vi "Resp.vi"(6 "Array 6":string[][](array[string]), 7 "Array":string[][](array[string]), 8 "Array 5":string[][](array[string]), 9 "Array 4":string[][](array[string]), 10 "Array 3":string[][](array[string]), 11 "Array 2":string[][](array[string])) -> (3 "output cluster":T1)   [LabVIEW 2014]
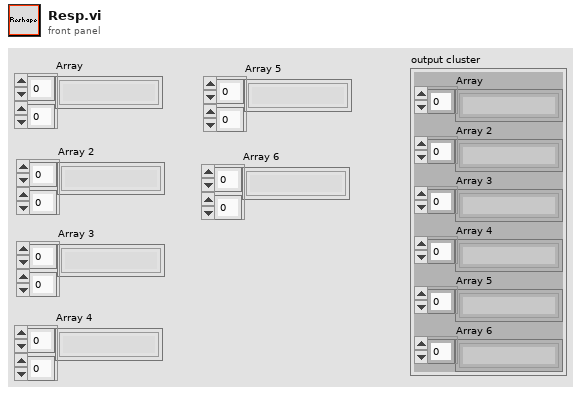
[diagram p1: front panel]
types:
  T1 = cluster{"Array":string[], "Array 2":string[], "Array 3":string[], "Array 4":string[], "Array 5":string[], "Array 6":string[]}
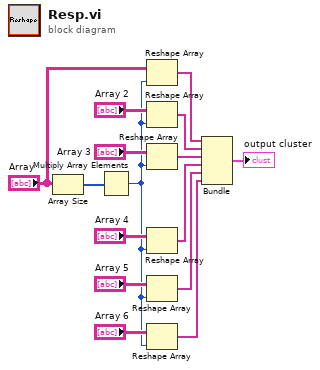
[diagram p0: block diagram]
diagram:
  n1 = Array Size(array="Array") -> (size(s)=w3:i32[])
  n2 = Multiply Array Elements(1:w3) -> (0:w2:i32)
  n3 = Reshape Array("Array", w2) -> (w10:string[])
  n4 = Reshape Array("Array 2", w2) -> (w9:string[])
  n5 = Reshape Array("Array 3", w2) -> (w8:string[])
  n6 = Reshape Array("Array 4", w2) -> (w7:string[])
  n7 = Reshape Array("Array 5", w2) -> (w6:string[])
  n8 = Reshape Array("Array 6", w2) -> (w5:string[])
  n9 = Bundle("Array"=w10, "Array 2"=w9, "Array 3"=w8, "Array 4"=w7, "Array 5"=w6, "Array 6"=w5) -> (→"output cluster":T1)  [unwired: 1 in]
